vi "ROSmsg_createAndWireClust.vi"(8 "error in (no error)":errorcluster, 10 "Terminals":refnum<vi>[](array[refnum]), 11 "Bundler in":refnum<vi>) -> (0 "error out":errorcluster, 3 "Cluster out":refnum<vi>)   [LabVIEW 2016]
doc: "Creates a cluster indicator"
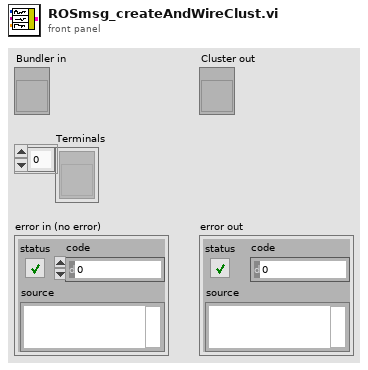
[diagram p1: front panel]
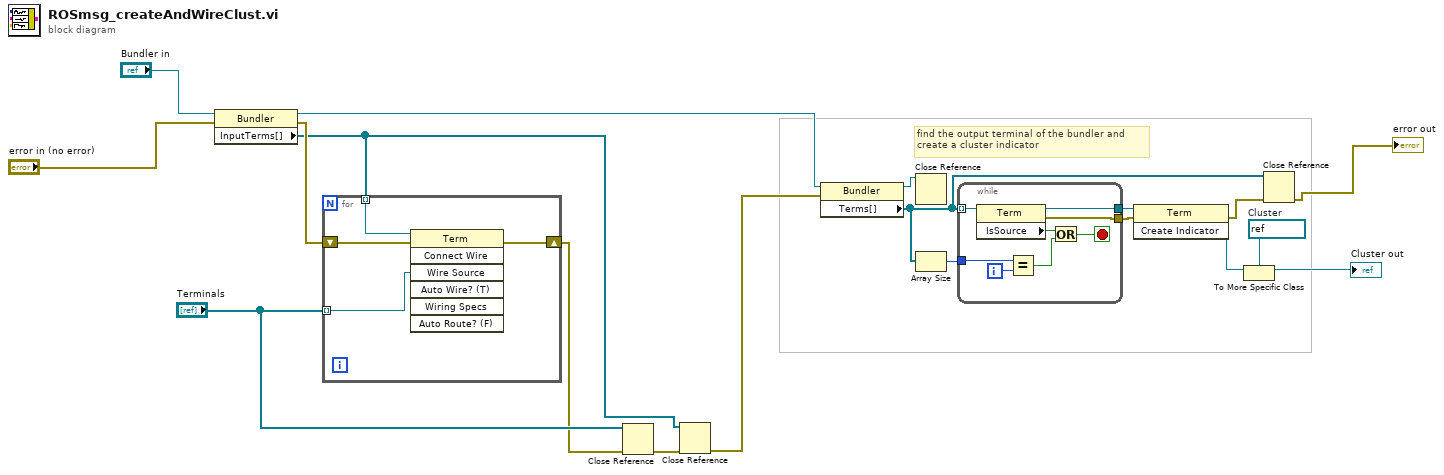
[diagram p0: block diagram]
diagram:
  w9 = refnum<vi> refnum  # Cluster
  # "find the output terminal of the bundler and \ncreate a cluster indicator"
  n1 = property class="Bundler"(reference="Bundler in", error in="error in (no error)") -> (reference out=w2:refnum<vi>, error out=w11:errorcluster, "InputTerms[]"=w8:refnum<vi>[])
  n2 = for {
    tunnel: w8 -> [w23] mode=indexing
    tunnel: "Terminals" -> [w22] mode=indexing
    shift-right: [w21] -> w6
    shift-left: w11 -> [w20]
    n3 = invoke class="Term" method="Connect Wire"(reference=w23, error in=w20, "Wire Source"=w22) -> (error out=w21:errorcluster)  [unwired: 4 in, 6 out]
  }
  n4 = Close Reference(reference="Terminals", error in (no error)=w6) -> (error out=w12:errorcluster)
  n5 = Close Reference(reference=w8, error in (no error)=w12) -> (error out=w13:errorcluster)
  n6 = property class="Bundler"(reference=w2, error in=w13) -> (reference out=w5:refnum<vi>, "Terms[]"=w16:refnum<vi>[])  [unwired: 1 out]
  n7 = Close Reference(reference=w5) -> ()  [unwired: 1 in, 1 out]
  n8 = Array Size(array=w16) -> (size(s)=w3:i32)
  n9 = while {
    tunnel: w16 -> [w31] mode=indexing
    tunnel: [w30] -> w4
    tunnel: w3 -> [w29]
    tunnel: [w24] -> w19
    i -> [w28]
    stop <- w25 stop-if-true
    n10 = property class="Term"(reference=w31) -> (reference out=w30:refnum<vi>, error out=w24:errorcluster, "IsSource"=w27:bool)  [unwired: 1 in]
    n11 = Equal?(x=w29, y=w28) -> (x = y?=w26:bool)
    n12 = Or(x=w27, y=w26) -> (x .or. y?=w25:bool)
  }
  n13 = invoke class="Term" method="Create Indicator"(reference=w4, error in=w19) -> (error out=w15:errorcluster, "Create Indicator"=w14:refnum<vi>)  [unwired: 1 in, 1 out]
  n14 = To More Specific Class(target class=w9, reference=w14) -> (specific class reference=→"Cluster out":refnum<vi>)  [unwired: 1 in, 1 out]
  n15 = Close Reference(reference=w16, error in (no error)=w15) -> (error out=→"error out":errorcluster)
